vi "DriveDistanceYAdvanced.vi"(2 "Parameter String":string, 3 "Reinit":bool) -> (0 "Error Out":errorcluster, 1 "Increment":bool)   [LabVIEW 2020]
doc: "The swerve drive base will translate in the field-centric Y direction at a speed specified by the joystick command. This is a \"medium smart\" algorithm, there is an orientation lock and overshoot prevention. Any complex or critical translations should be handled using either the Path Follower or auto-targeting. \n\nParameters:\n1. relative travel distance in the field-centric Y direction --> (in) [-323,323]\n2. undershoot error- the number of inches under the goal allowed --> (in) [0,323]\n3. overshoot error- the number of inches over the goal allowed --> (in) [0,323]\n4. timeout -->(ms) -1 to ignore [-1,15000]"
uses:
  SafeParser_Float.vi
  SafeParser_Integer.vi
  drivercommands.vi
  sensordata.vi
  autonomousinfo.vi
panel:
  in  "PID Tuning Drive":T1={"Kp"=0.01, "Ki"=0.0, "Kd"=0.0, "N-Diff"=10, "N-Int"=20, "Int Error Window"=0.5, "Max Ouput"=1.0, "Min Output"=-1.0} {"Int Error Window" min=0.0; "N-Int" min=2; "N-Diff" min=2; "Kd" min=0.0; "Ki" min=0.0; "Kp" min=0.0}
  out "Drive PID":T2(graph)
  out "Rotation PID":T2(graph)
  in  "Plots?":bool
  in  "Time in Range (ms)":u32=1000
  in  "PID Tuning Rotation":T1={"Kp"=0.007, "Ki"=0.03, "Kd"=0.001, "N-Diff"=5, "N-Int"=10, "Int Error Window"=30.0, "Max Ouput"=1.0, "Min Output"=-1.0} {"Int Error Window" min=0.0; "N-Int" min=2; "N-Diff" min=2; "Kd" min=0.0; "Ki" min=0.0; "Kp" min=0.0}
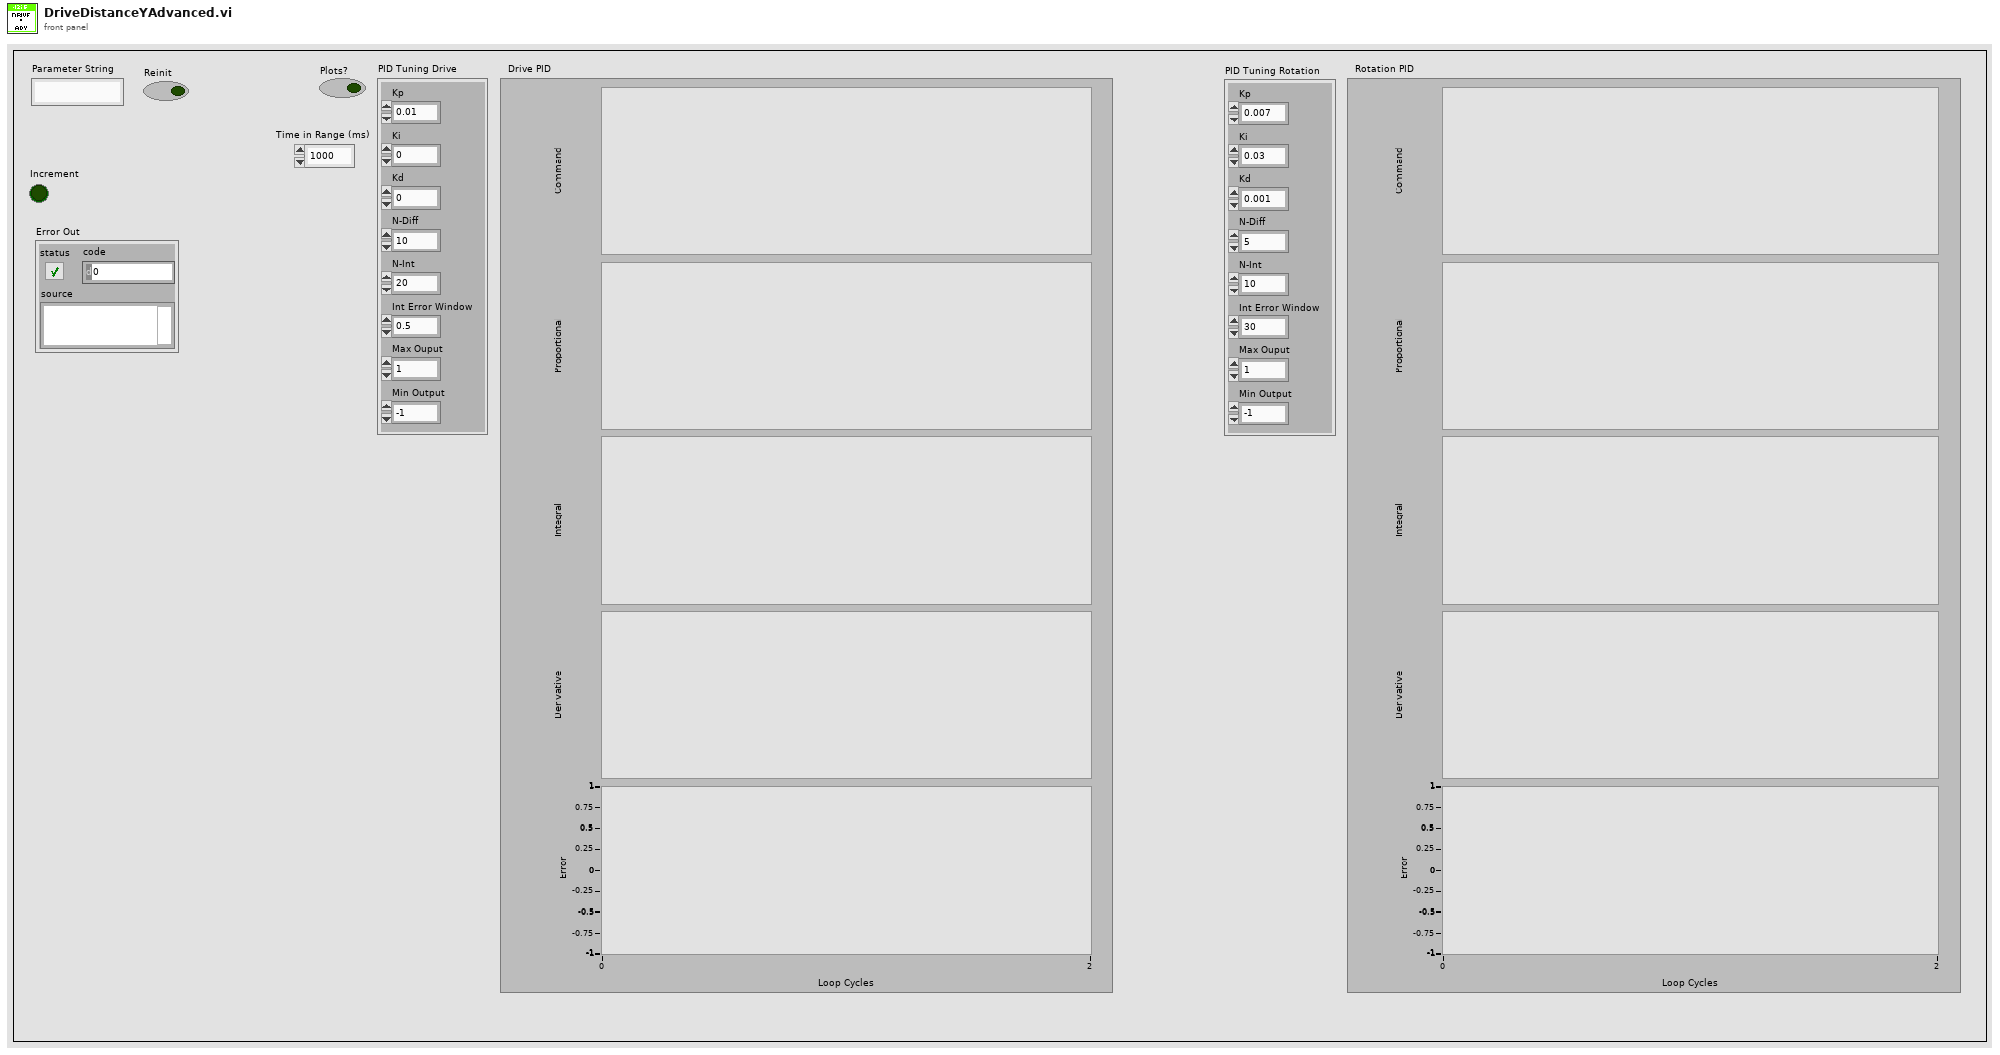
[diagram p1: front panel]
types:
  T1 = cluster{"Kp":dbl, "Ki":dbl, "Kd":dbl, "N-Diff":i32, "N-Int":i32, "Int Error Window":dbl, "Max Ouput":dbl, "Min Output":dbl}
  T2 = cluster{"Command":dbl, "Proportional":dbl, "Integral":dbl, "Derivative":dbl, "Goal":dbl}
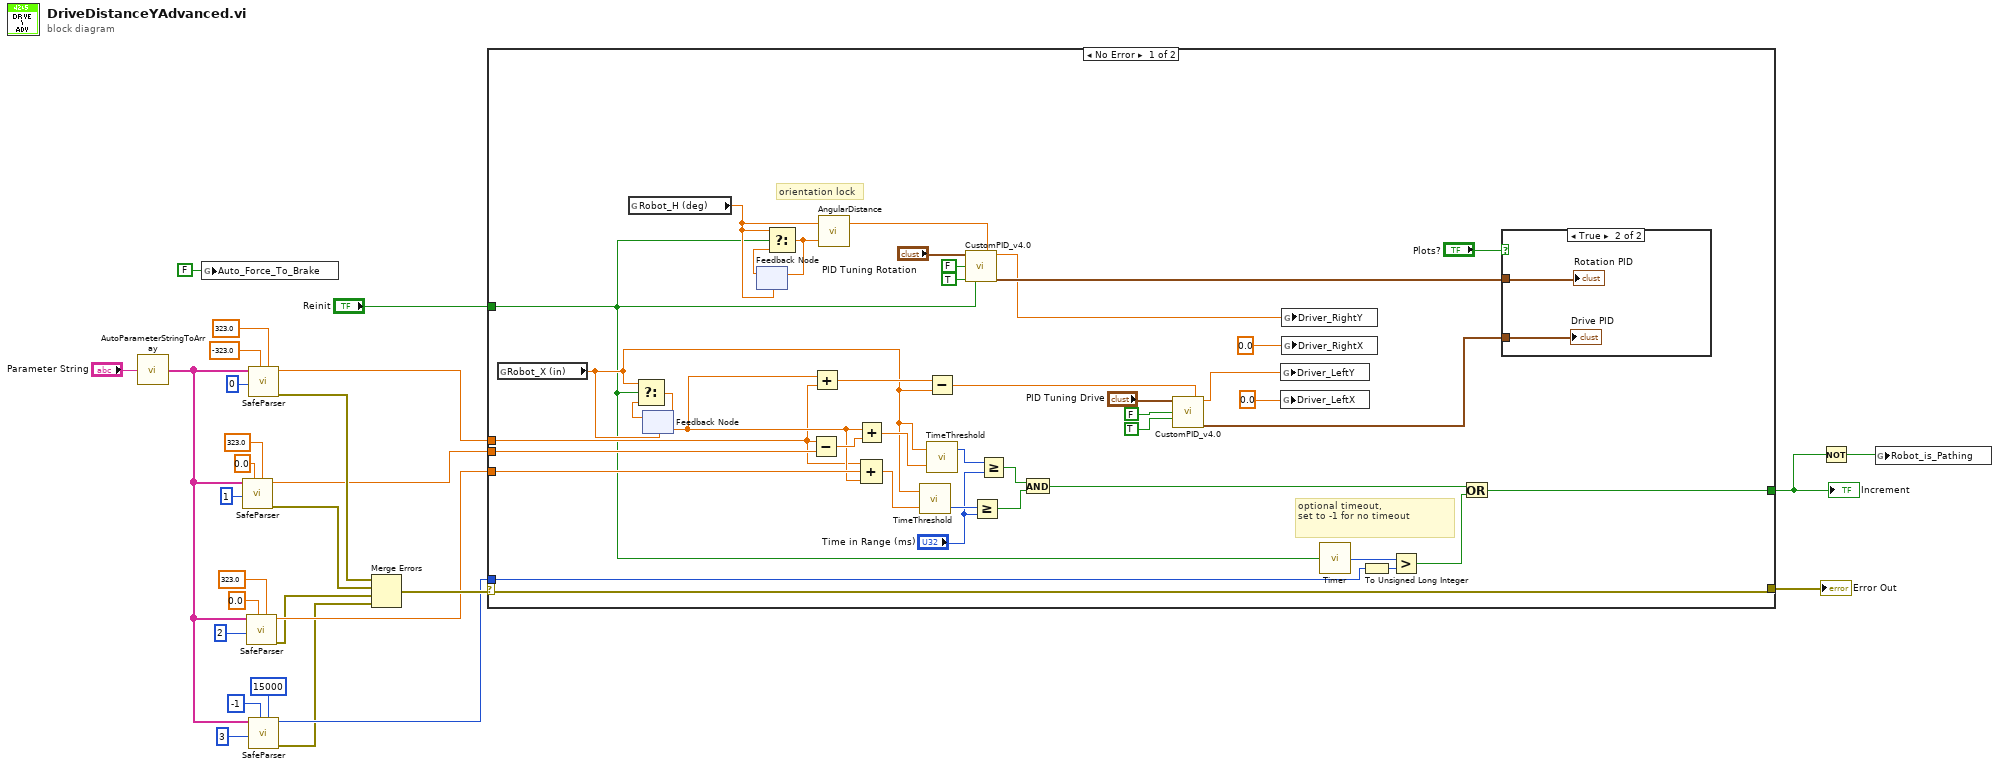
[diagram p0: block diagram]
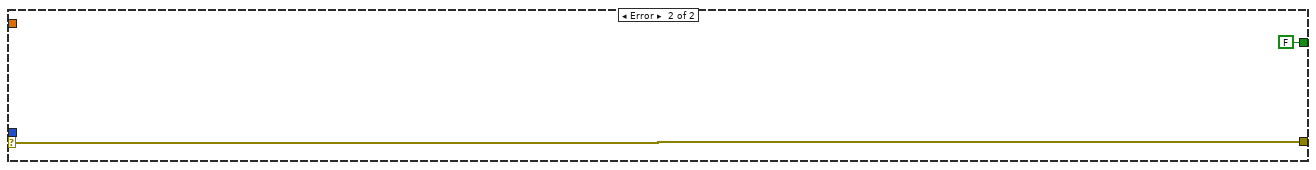
[diagram p3: hidden frame]
diagram:
  n1 = call "AutoParameterStringToArray.vi"("Parameter String"="Parameter String") -> ("Parsed Parameters"=w7:string[])
  n2 = global write "autonomousinfo.vi" "Auto_Force_To_Brake"(FALSE ("Auto_Force_To_Brake")) -> ()
  n3 = call-poly "SafeParser.vi"("Maximum"=323.0, "Minimum"=0.0, "Array Index"=1 ("Parameter Index"), "String Array"=w7) -> ("Error Out"=w21:errorcluster, "Typecast  Value"=w18:dbl)  [unwired: 6 in]
  n4 = call-poly "SafeParser.vi"("Maximum"=323.0, "Minimum"=0.0, "Array Index"=2 ("Parameter Index"), "String Array"=w7) -> ("Error Out"=w11:errorcluster, "Typecast  Value"=w12:dbl)  [unwired: 6 in]
  n5 = call-poly "SafeParser.vi"("Maximum"=323.0, "Minimum"=-323.0, "Array Index"=0 ("Parameter Index"), "String Array"=w7) -> ("Error Out"=w20:errorcluster, "Typecast  Value"=w10:dbl)  [unwired: 6 in]
  n6 = call-poly "SafeParser.vi"("Maximum"=15000, "Minimum"=-1, "Array Index"=3 ("Parameter Index"), "String Array"=w7) -> ("Error Out"=w4:errorcluster, "Typecast  Value"=w5:i32)  [unwired: 6 in]
  n7 = Merge Errors(w20, w21, w11, w4) -> (w19:errorcluster)
  n8 = case shown="No Error" w19 {
    selector: w19 -> [w68 w73]
    tunnel: [w31 FALSE] -> w2
    tunnel: "Reinit" -> [w35 _]
    tunnel: [w68 w73] -> w27
    tunnel: w10 -> [w59 _]
    tunnel: w18 -> [w63 _]
    tunnel: w12 -> [w64 _]
    tunnel: w5 -> [w34 _]
    frame No Error {
      # "optional timeout,\nset to -1 for no timeout"
      # "orientation lock"
      n9 = global read "sensordata.vi" "Robot_X (in)"() -> (w48:dbl)
      n10 = global read "sensordata.vi" "Robot_H (deg)"() -> (w46:dbl)
      n11 = feedback #1(w48) -> (w62:dbl)
      n12 = Select(t=w48, s=w35, f=w62) -> (s? t:f=w60:dbl)
      n13 = feedback-in #1(w60) -> ()
      n14 = feedback #2(w46) -> (w44:dbl)
      n15 = Select(t=w46, s=w35, f=w44) -> (s? t:f=w45:dbl)
      n16 = feedback-in #2(w45) -> ()
      n17 = Subtract(x=w59, y=w63) -> (x-y=w61:dbl)
      n18 = Add(x=w60, y=w59) -> (x+y=w58:dbl)
      n19 = call "AngularDistance.vi"("Goal Angle (deg) [0,360]"=w45, "Current Angle (deg) [-Inf,+Inf]"=w46) -> ("Signed Angular Distance (deg) [-180,+180]"=w38:dbl)  [unwired: 1 out]
      n20 = Add(x=w60, y=w61) -> (x+y=w52:dbl)
      n21 = Compound Arithmetic op=ADD(w59, w64, w60) -> (w55:dbl)
      n22 = call "TimeThreshold.vi"("Threshold"=w55, "Current Value"=w48) -> ("Time Below Threshold (ms)"=w54:u32)  [unwired: 1 out]
      n23 = Subtract(x=w58, y=w48) -> (x-y=w47:dbl)
      n24 = call "TimeThreshold.vi"("Threshold"=w52, "Current Value"=w48) -> ("Time Above Threshold (ms)"=w51:u32)  [unwired: 1 out]
      n25 = call "CustomPID_v4.0.vi"("PID Tuning Parameters"="PID Tuning Rotation", "Custom Error Calculation"=w38, "Reset on Goal Change ?"=FALSE, "Use Custom Error Calculation ?"=TRUE, "Reinit"=w35) -> ("Command"=w39:dbl, "Controller Summary"=w40:T2)  [unwired: 7 in, 2 out]
      n26 = Greater Or Equal?(x=w54, y="Time in Range (ms)") -> (x >= y?=w53:bool)
      n27 = Greater Or Equal?(x=w51, y="Time in Range (ms)") -> (x >= y?=w49:bool)
      n28 = And(x=w49, y=w53) -> (x .and. y?=w33:bool)
      n29 = call "CustomPID_v4.0.vi"("PID Tuning Parameters"="PID Tuning Drive", "Custom Error Calculation"=w47, "Reset on Goal Change ?"=FALSE, "Use Custom Error Calculation ?"=TRUE) -> ("Command"=w30:dbl, "Controller Summary"=w56:T2)  [unwired: 8 in, 2 out]
      n30 = global write "drivercommands.vi" "Driver_LeftY"(w30) -> ()
      n31 = global write "drivercommands.vi" "Driver_LeftX"(0.0 ("Driver_LeftX")) -> ()
      n32 = global write "drivercommands.vi" "Driver_RightY"(w39) -> ()
      n33 = global write "drivercommands.vi" "Driver_RightX"(0.0 ("Driver_RightX")) -> ()
      n34 = call "Timer.vi"("Reset Timer"=w35) -> ("Time (ms)"=w36:u32)
      n35 = To Unsigned Long Integer(number=w34) -> (unsigned 32bit integer=w37:u32)
      n36 = Greater?(x=w36, y=w37) -> (0:w32:bool)
      n37 = Or(x=w33, y=w32) -> (x .or. y?=w31:bool)
      n38 = case shown="True" "Plots?" {
        tunnel: w56 -> [_ w71]
        tunnel: w40 -> [_ w70]
        frame False {
        }
        frame True {
          "Drive PID" <- w71
          "Rotation PID" <- w70
        }
      }
    }
    frame Error {
    }
  }
  "Increment" <- w2
  "Error Out" <- w27
  n39 = Not(x=w2) -> (.not. x?=w3:bool)
  n40 = global write "autonomousinfo.vi" "Robot_is_Pathing"(w3) -> ()
